vi "Find Broken VIs in a Folder.vi"(8 "error in (no error)":errorcluster, 11 "Directory Path":path) -> (0 "error out":errorcluster, 3 "Broken VIs":path[](array[path]))   [LabVIEW 2016, in "SLL Scripting.lvlib"]
doc: "This VI can be used to find the list of broken VIs in a folder. \n\nKindly note that this would also return VIs which are of higher LabVIEW version than the currently used LabVIEW version."
uses:
  SLL Scripting.lvlib
panel:
  out "Progress":i32
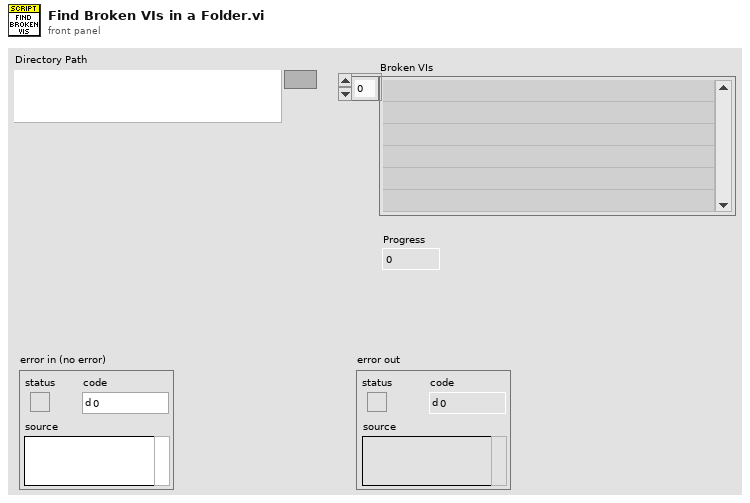
[diagram p1: front panel]
types:
  T1 = enum32{"Bad", "Idle", "Run top level", "Running"}
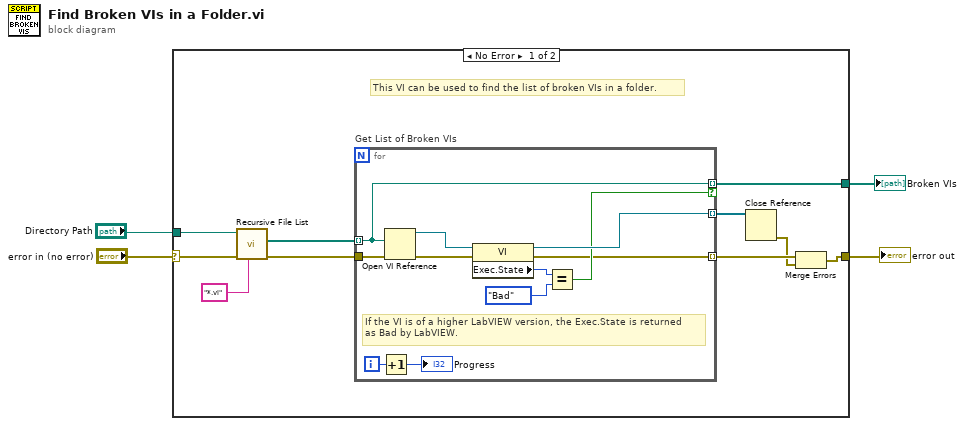
[diagram p0: block diagram]
diagram:
  n1 = case shown="No Error" "error in (no error)" {
    selector: "error in (no error)" -> [w9 w26]
    tunnel: "Directory Path" -> [w13 _]
    tunnel: [w10 _] -> w3
    tunnel: [w5 w26] -> w1
    frame No Error {
      # "This VI can be used to find the list of broken VIs in a folder."
      n2 = call <vilib>:"Recursive File List.vi"("pattern"="*.vi", "error in (no error)"=w9, "Folder Path"=w13) -> ("error out"=w8:errorcluster, "All Files in Dir"=w11:path[])  [unwired: 4 in, 3 out]
      n3 = for "Get List of Broken VIs" {
        tunnel: [w22] -> w14 mode=indexing
        tunnel: w11 -> [w21] mode=indexing
        tunnel: [w21] -> w10 mode=indexing if=w20
        tunnel: w8 -> [w19]
        tunnel: [w17] -> w7 mode=indexing
        i -> [w16]
        # "If the VI is of a higher LabVIEW version, the Exec.State is returned\nas Bad by LabVIEW."
        n4 = Increment(x=w16) -> (x+1=→"Progress":i32)
        n5 = Open VI Reference(vi path=w21, error in (no error)=w19) -> (vi reference=w25:refnum<vi>, error out=w18:errorcluster)  [unwired: 4 in]
        n6 = property class="VI"(reference=w25, error in=w18) -> (reference out=w22:refnum<vi>, error out=w17:errorcluster, "Exec.State"=w24:T1)
        n7 = Equal?(x=w24, y=T1."Bad" ("Execution:State")) -> (x = y?=w20:bool)
      }
      n8 = Close Reference(reference=w14) -> (error out=w6:errorcluster)  [unwired: 1 in]
      n9 = Merge Errors(w7, w6) -> (w5:errorcluster)
    }
    frame Error {
    }
  }
  "error out" <- w1
  "Broken VIs" <- w3
